vi "Read Actor Core Reference.vi"(11 "IViewable In":refnum<class "IViewable.lvclass">) -> (2 "Actor Core Refnum":refnum<vi>, 3 "IViewable Out":refnum<class "IViewable.lvclass">)   [LabVIEW 2017, in "IViewable.lvlib" / "IViewable.lvclass"]
doc: "<License>\nCopyright © 2017 Composed Systems, LLC | All rights reserved\nwww.composed.io\n\nAuthor: Ethan Stern <ethan.stern@composed.io>\n\nThis software is provided \"AS IS\" WITHOUT WARRANTIES, either express or implied, AND IS FOR EDUCATIONAL PURPOSES ONLY.\n</License>"
uses:
  IViewable.lvclass
  IViewable.lvclass/IViewable.ctl
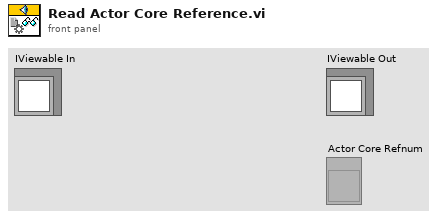
[diagram p1: front panel]
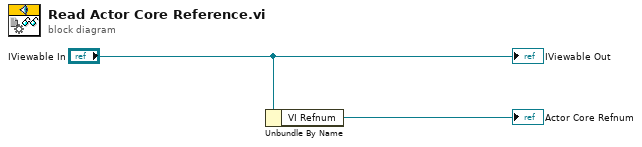
[diagram p0: block diagram]
diagram:
  n1 = Unbundle By Name("IViewable In") -> ("VI Refnum"=→"Actor Core Refnum":refnum<vi>)
  "IViewable Out" <- "IViewable In"
